vi "Add User Comment.vi"(8 "error in":errorcluster, 11 "Console Log in":refnum<class "Console Log.lvclass">) -> (0 "error out":errorcluster, 3 "Console Log out":refnum<class "Console Log.lvclass">)   [LabVIEW 2011, in "Console Log.lvclass"]
uses:
  Console Log.lvclass
  Console Log.lvclass/Console Log.ctl
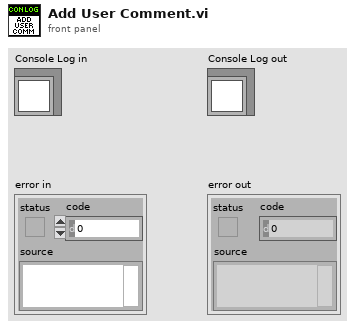
[diagram p1: front panel]
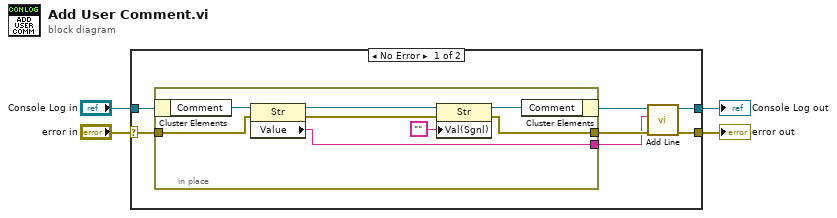
[diagram p0: block diagram]
diagram:
  n1 = case shown="No Error" "error in" {
    selector: "error in" -> [w10 w21]
    tunnel: [w5 w21] -> w3
    tunnel: [w8 w20] -> w1
    tunnel: "Console Log in" -> [w11 w20]
    frame No Error {
      n2 = in-place {
        in-place-border: [w14] -> w7
        in-place-border: w10 -> [w13]
        in-place-border: [w12] -> w6
        n3 = in-place-cluster #1(w11) -> ("Comment"=w19:refnum<vi>)
        n4 = property class="Str"(reference=w19, error in=w13) -> (reference out=w18:refnum<vi>, error out=w15:errorcluster, "Value"=w12:string)
        n5 = property class="Str"(reference=w18, error in=w15, "Val(Sgnl)"="") -> (reference out=w17:refnum<vi>, error out=w14:errorcluster)
        n6 = in-place-cluster #1("Comment"=w17) -> (w9:refnum<class "Console Log.lvclass">)
      }
      n7 = call "Add Line.vi"("error in"=w7, "String"=w6, "Console Log in"=w9) -> ("error out"=w5:errorcluster, "Console Log out"=w8:refnum<class "Console Log.lvclass">)  [unwired: 7 in]
    }
    frame Error {
    }
  }
  "error out" <- w3
  "Console Log out" <- w1
